vi "To Byte Array (EEPROM Calibration Header).vi"(1 "EEPROM Calibration Header":T1 {"Checksum" format="%x"}) -> (0 "byte array out":u8[](array[numeric]) format="%x")   [LabVIEW 2013]
uses:
  <instrlib>/ni579x/Config/v1/Shared/Types/EEPROM/ni579x EEPROM Calibration Header.ctl
  <instrlib>/ni579x/Config/v1/Shared/Conversions/To Byte Array (U32).vi
  <instrlib>/ni579x/Config/v1/Shared/Conversions/To Byte Array (F32).vi
  <instrlib>/ni579x/Config/v1/Shared/Conversions/To Byte Array (LV Timestamp).vi
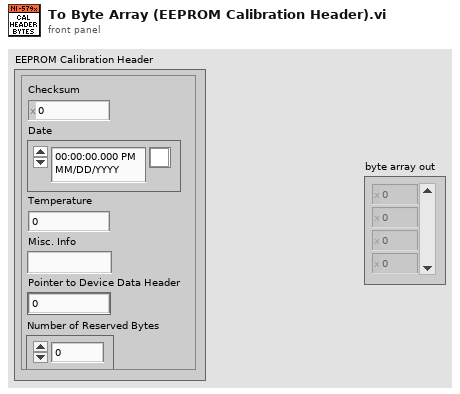
[diagram p1: front panel]
types:
  T1 = typedef "ni579x EEPROM Calibration Header.ctl" = cluster{"Checksum":u32, "Date":timestamp, "Temperature":sgl, "Misc. Info":string, "Pointer to Device Data Header":u32, "Number of Reserved Bytes":i32}
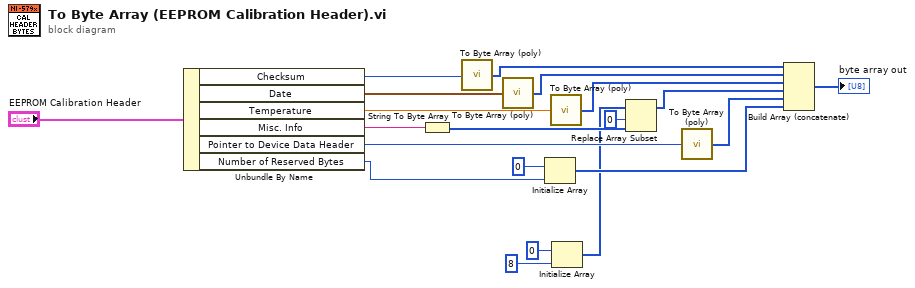
[diagram p0: block diagram]
diagram:
  n1 = Unbundle By Name("EEPROM Calibration Header") -> ("Checksum"=w16:u32, "Date"=w17:timestamp, "Temperature"=w15:sgl, "Misc. Info"=w5:string, "Pointer to Device Data Header"=w14:u32, "Number of Reserved Bytes"=w12:i32)
  n2 = String To Byte Array(string=w5) -> (unsigned byte array=w4:u8[])
  n3 = call-poly <instrlib>:"To Byte Array (poly).vi"("element in"=w16) -> ("byte array out"=w11:u8[])
  n4 = call-poly <instrlib>:"To Byte Array (poly).vi"("element in"=w17) -> ("byte array out"=w10:u8[])
  n5 = Initialize Array(u8 0, w12) -> (w7:u8[])
  n6 = call-poly <instrlib>:"To Byte Array (poly).vi"("element in"=w15) -> ("byte array out"=w9:u8[])
  n7 = Initialize Array(u8 0, 8 ("dimension size")) -> (w2:u8[])
  n8 = Replace Array Subset(array=w2, new element=w4, index=0) -> (w3:u8[])
  n9 = call-poly <instrlib>:"To Byte Array (poly).vi"("element in"=w14) -> ("byte array out"=w8:u8[])
  n10 = Build Array (concatenate)(w11, w10, w9, w3, w8, w7) -> (→"byte array out":u8[])
